vi "Aero_Tunnel_Server.vi"() -> ()   [LabVIEW 2010]
uses:
  Controls/Post_Process.ctl
  Globals/Meas_global.vi
panel:
  in  "Quit":bool
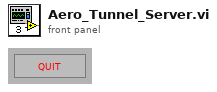
[diagram p1: front panel]
types:
  T1 = typedef "Post_Process.ctl" = enum16{"Take New Data", "Post Process Raw Data File"}
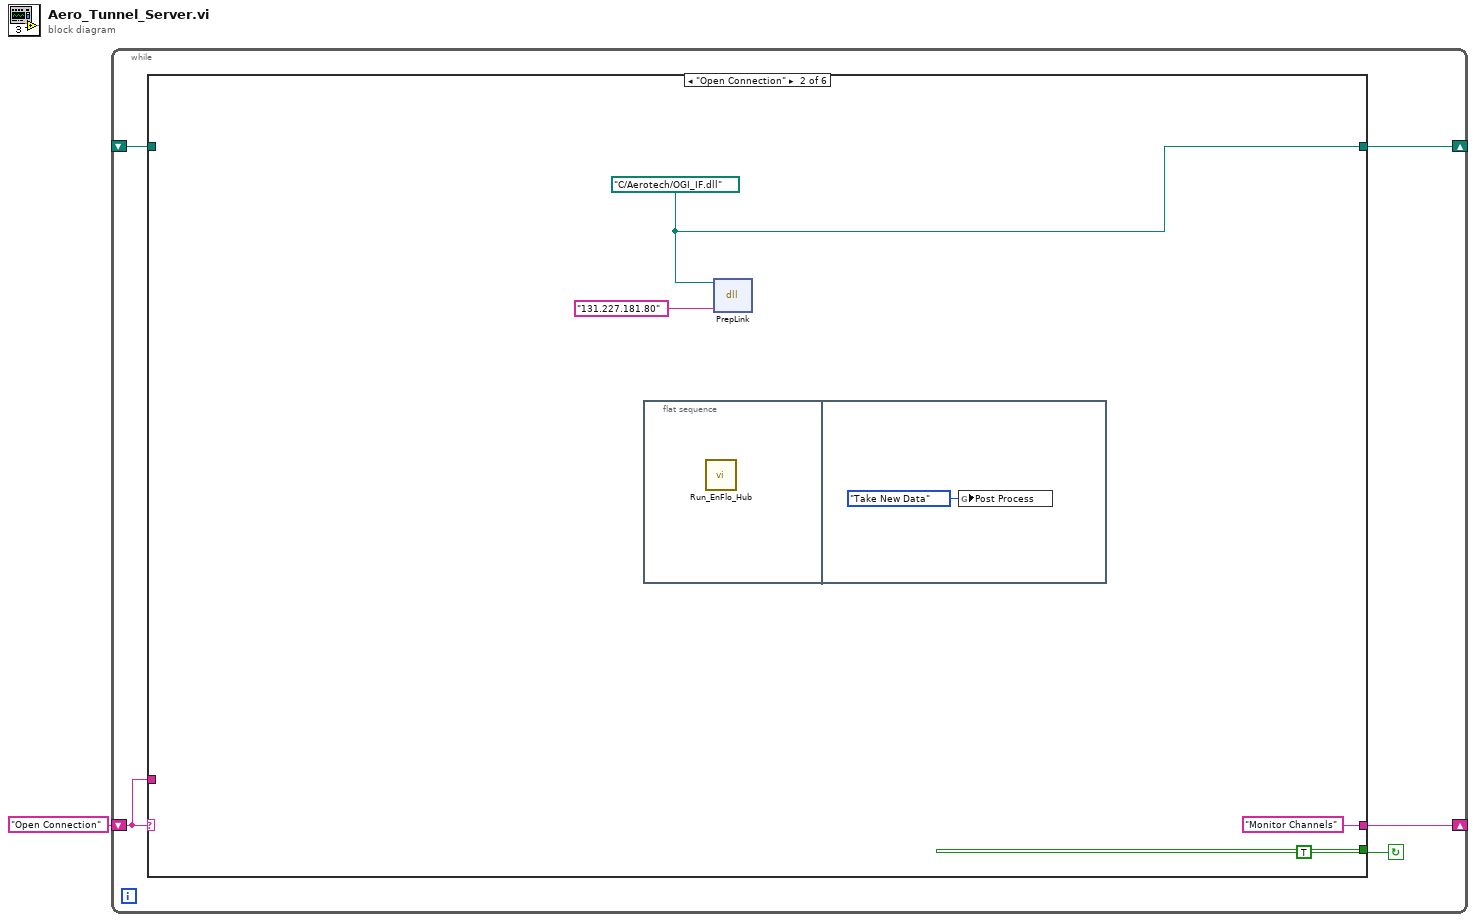
[diagram p0: block diagram]
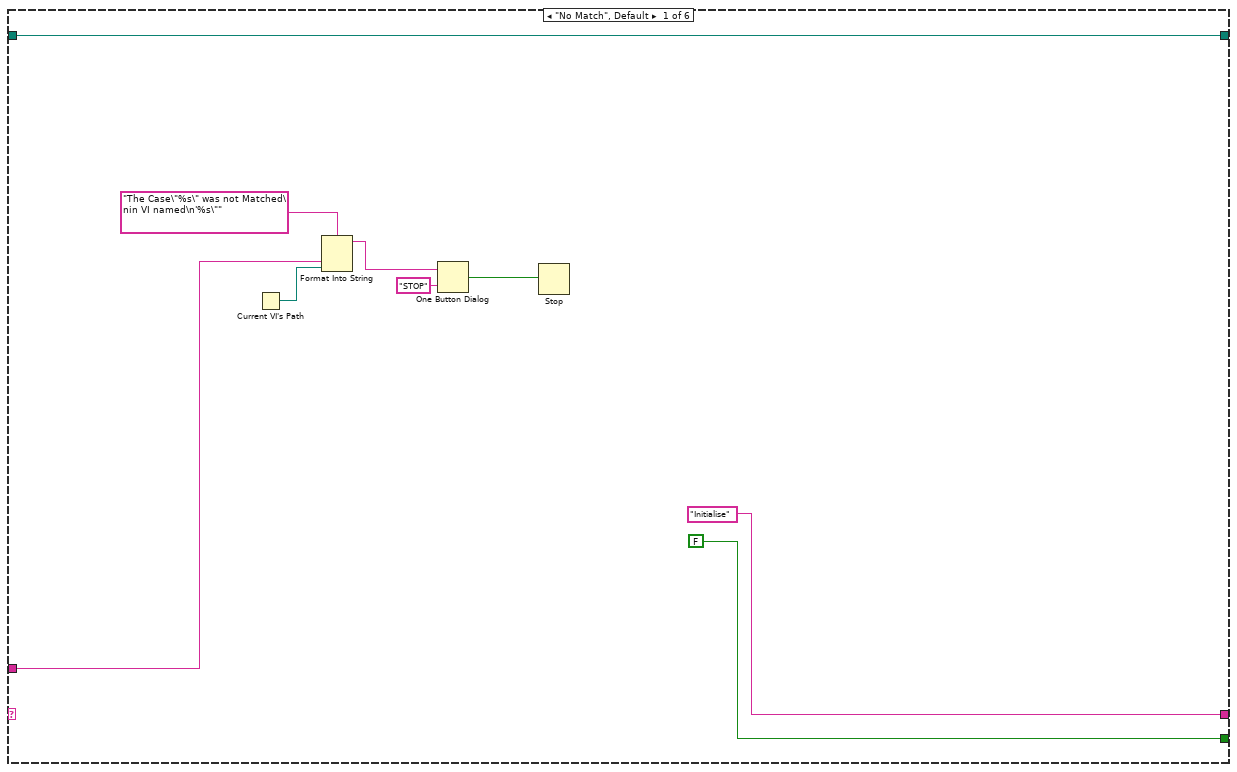
[diagram p2: hidden frame]
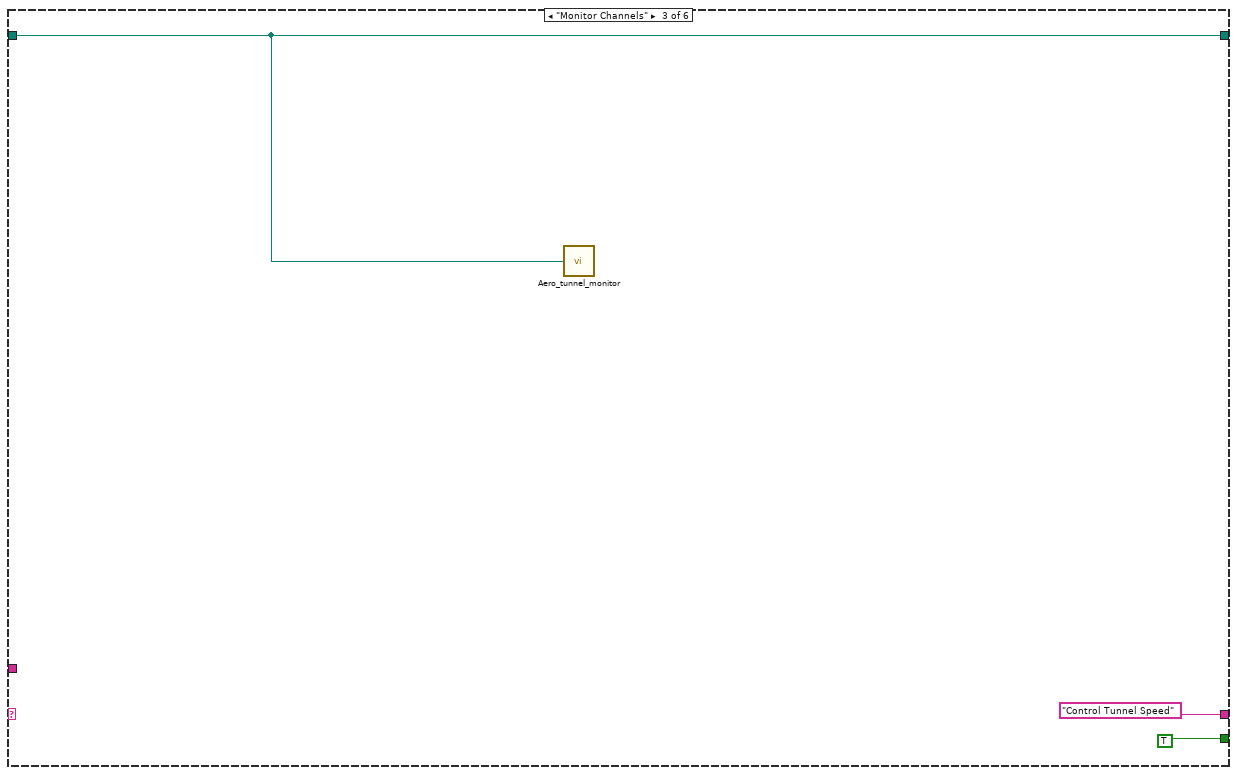
[diagram p3: hidden frame]
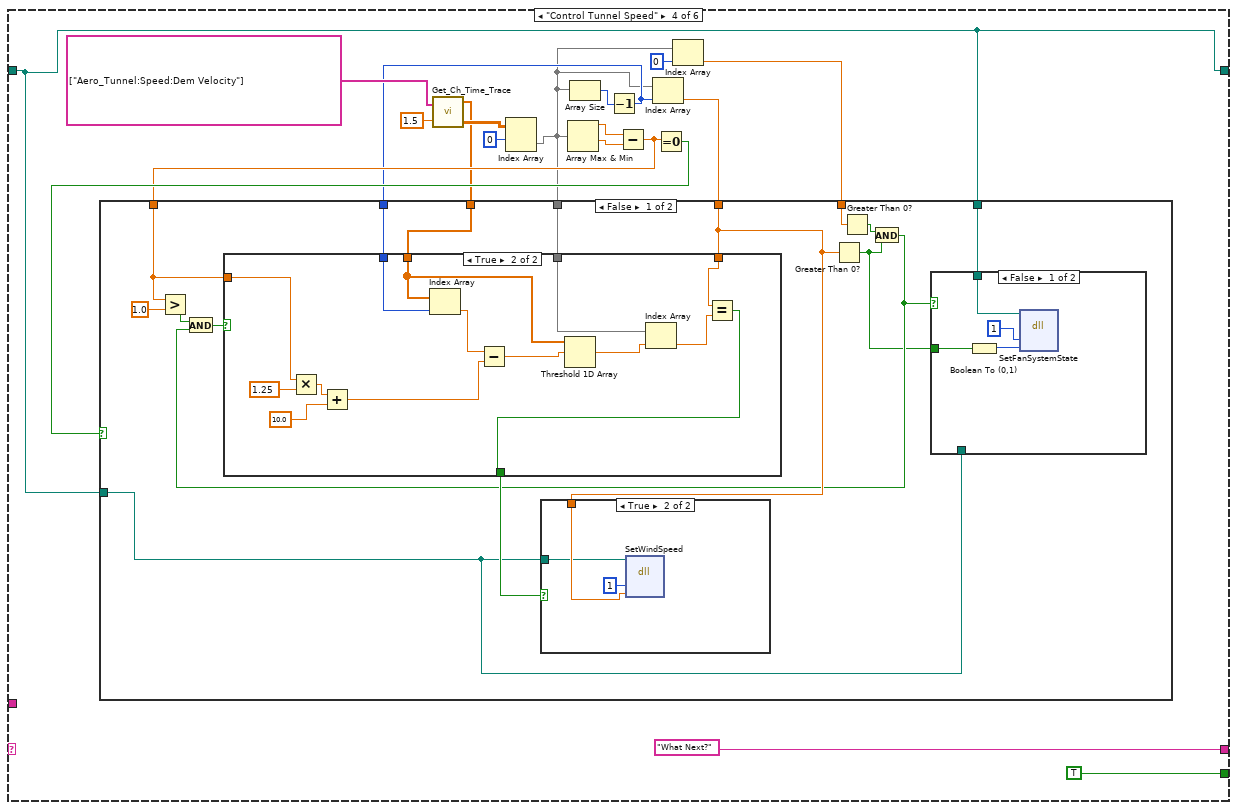
[diagram p4: hidden frame]
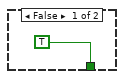
[diagram p7: hidden frame]
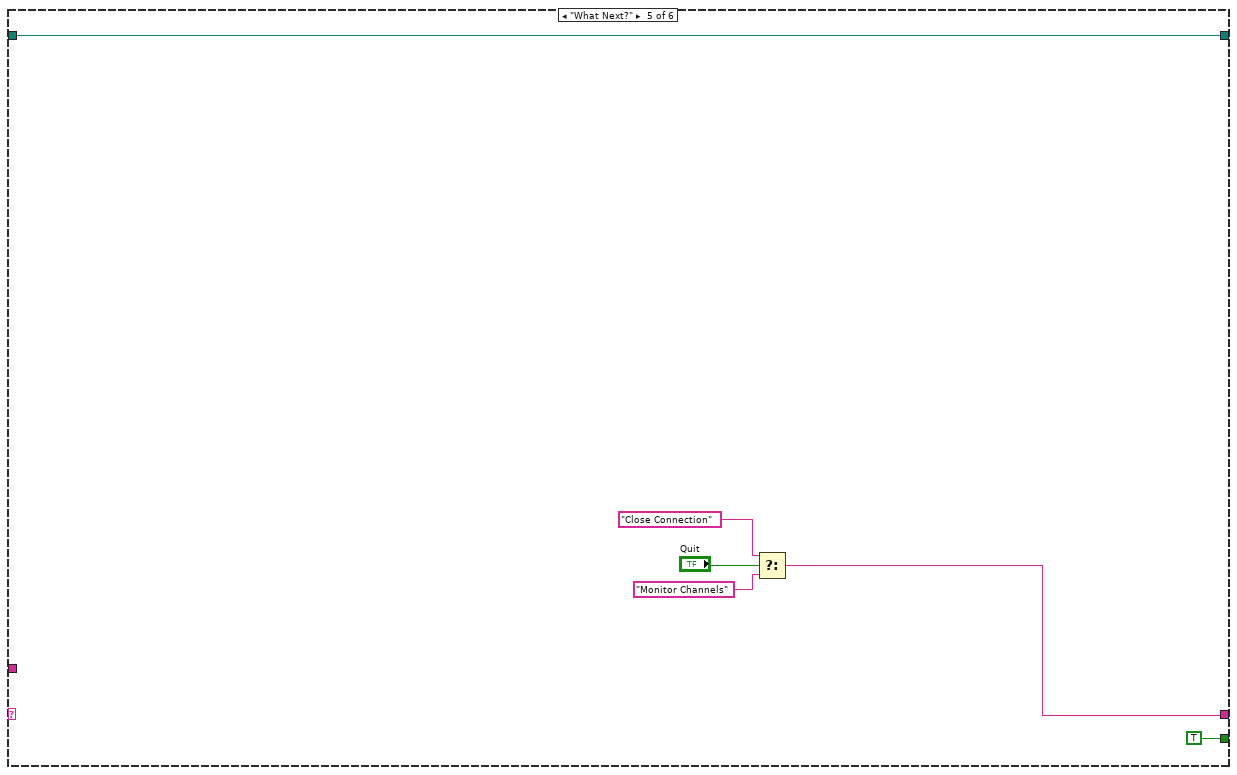
[diagram p9: hidden frame]
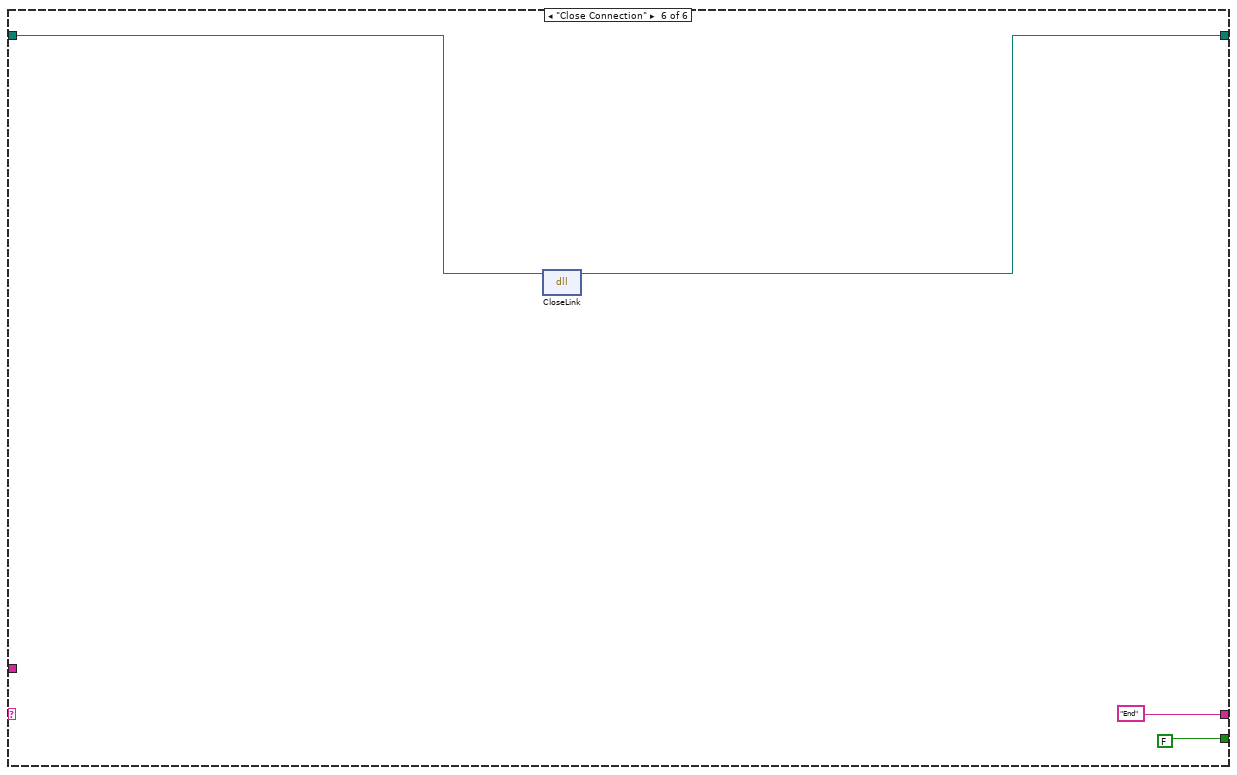
[diagram p10: hidden frame]
diagram:
  n1 = while {
    shift-left: "Open Connection" -> [w4]
    shift-right: [w5] -> _
    shift-right: [w3] -> _
    shift-left: _ -> [w2]
    stop <- w6 continue-if-true
    n2 = case shown="\"Open Connection\"" w4 {
      tunnel: [FALSE TRUE TRUE TRUE TRUE FALSE] -> w6
      tunnel: ["Initialise" "Monitor Channels" "Control Tunnel Speed" "What Next?" w80 "End"] -> w5
      tunnel: w4 -> [w10 _ _ _ _ _]
      tunnel: [w7 w16 w21 w24 w79 w85] -> w3
      tunnel: w2 -> [w7 _ w21 w24 w79 w86]
      frame "No Match", Default {
        n3 = Current VI's Path() -> (path=w9:path)
        n4 = Format Into String(format string="The Case\"%s\" was not Matched\nin VI named\n'%s\"" ("Format String"), w10, w9) -> (resulting string=w13:string)  [unwired: 2 in, 1 out]
        n5 = One Button Dialog(message=w13, button name ("OK")="STOP") -> (true=w11:bool)
        n6 = Stop(stop? (T)=w11) -> ()
      }
      frame "Open Connection" {
        w16 = path "C:/Aerotech/OGI_IF.dll" ("path in")
        n7 = flat-sequence {
          frame #0 {
            n8 = call "Run_EnFlo_Hub.vi"() -> ()  [unwired: 8 out]
          }
          frame #1 {
            n9 = global write "Meas_global.vi" "Post Process"(Post_Process."Take New Data" ("Post Process")) -> ()
          }
        }
        n10 = dll-call lib="C:/Aerotech/Drivers/OGI_IF.dll" fn="PrepLink"(path in=w16, "IPAddress"="131.227.181.80") -> ()  [unwired: 2 in, 4 out]
      }
      frame "Monitor Channels" {
        n11 = call "Aero_tunnel_monitor.vi"("path in"=w21) -> ()  [unwired: 1 out]
      }
      frame "Control Tunnel Speed" {
        n12 = call "Get_Ch_Time_Trace.vi"("Desired Ch Names"=string[] ["Aero_Tunnel:Speed:Dem Velocity"] ("ADAM Ch Names"), "History Length (mins)"=1.5) -> ("Centre Times"=w29:dbl[], "Output array"=w36:dbl[][])  [unwired: 1 out]
        n13 = Index Array(array=w36, index (row)=0 ("index")) -> (element=w26:dbl[])  [unwired: 1 in]
        n14 = Array Max & Min(array=w26) -> (max value=w35:dbl, min value=w34:dbl)  [unwired: 2 out]
        n15 = Array Size(array=w26) -> (size(s)=w31:i32)
        n16 = Decrement(x=w31) -> (x-1=w28:i32)
        n17 = Subtract(x=w35, y=w34) -> (x-y=w32:dbl)
        n18 = Index Array(array=w26, index=w28) -> (element=w30:dbl)
        n19 = Equal To 0?(x=w32) -> (x = 0?=w33:bool)
        n20 = Index Array(array=w26, index=0) -> (element=w25:dbl)
        n21 = case shown="False" w33 {
          tunnel: w32 -> [w53 _]
          tunnel: w24 -> [w43 _]
          tunnel: w30 -> [w48 _]
          tunnel: w29 -> [w55 _]
          tunnel: w28 -> [w54 _]
          tunnel: w26 -> [w52 _]
          tunnel: w25 -> [w47 _]
          tunnel: w24 -> [w42 _]
          frame False {
            n22 = Greater?(x=w53, y=1.0) -> (0:w50:bool)
            n23 = Greater Than 0?(x=w48) -> (x > 0?=w44:bool)
            n24 = Greater Than 0?(x=w47) -> (x > 0?=w46:bool)
            n25 = And(x=w46, y=w44) -> (x .and. y?=w45:bool)
            n26 = And(x=w50, y=w45) -> (x .and. y?=w49:bool)
            n27 = case shown="True" w49 {
              tunnel: w48 -> [_ w67]
              tunnel: w55 -> [_ w71]
              tunnel: w54 -> [_ w78]
              tunnel: w53 -> [_ w76]
              tunnel: w52 -> [_ w69]
              tunnel: [TRUE w65] -> w51
              frame False {
              }
              frame True {
                n28 = Multiply(x=w76, y=1.25) -> (x*y=w75:dbl)
                n29 = Add(x=w75, y=10.0) -> (x+y=w72:dbl)
                n30 = Index Array(array=w71, index=w78) -> (element=w73:dbl)
                n31 = Subtract(x=w73, y=w72) -> (x-y=w70:dbl)
                n32 = Threshold 1D Array(2:w70, 3:w71) -> (0:w68:dbl)  [unwired: 1 out]
                n33 = Index Array(array=w69, index=w68) -> (element=w66:dbl)
                n34 = Equal?(x=w67, y=w66) -> (x = y?=w65:bool)
              }
            }
            n35 = case shown="True" w51 {
              tunnel: w48 -> [_ w62]
              tunnel: w43 -> [_ w61]
              frame False {
              }
              frame True {
                n36 = dll-call lib="C:/Aerotech/Drivers/OGI_IF.dll" fn="SetWindSpeed"(path in=w61, "Enable"=1, "NewWindSpeed"=w62) -> ()  [unwired: 4 in, 3 out]
              }
            }
            n37 = case shown="False" w45 {
              tunnel: w44 -> [w60 _]
              tunnel: w43 -> [_ _]
              tunnel: w42 -> [w57 _]
              frame False {
                n38 = Boolean To (0,1)(Boolean=w60) -> (0, 1=w58:i16)
                n39 = dll-call lib="C:/Aerotech/Drivers/OGI_IF.dll" fn="SetFanSystemState"(path in=w57, "Enable"=1, "Fan ONOFF"=w58) -> ()  [unwired: 3 in, 4 out]
              }
              frame True {
              }
            }
          }
          frame True {
          }
        }
      }
      frame "What Next?" {
        n40 = Select(t="Close Connection", s="Quit", f="Monitor Channels") -> (s? t:f=w80:string)
      }
      frame "Close Connection" {
        n41 = dll-call lib="C:/Aerotech/Drivers/OGI_IF.dll" fn="CloseLink"(path in=w86) -> (path out=w85:path)  [unwired: 2 in, 2 out]
      }
    }
  }
